vi "Add Items to Graph.vi"(5 "Force Skip? (F)":bool, 7 "Depth Limit (12)":i32=12, 9 "Parent Index (None)":i32=-1, 10 "Items":variant[](array[variant]), 11 "Graph In":T1[](array[typedef])) -> (3 "Graph":T1[](array[typedef]))   [LabVIEW 2016, in "Better Search.lvlib"]
uses:
  Better Search.lvlib
  Data Types/Type Reflection Item.ctl
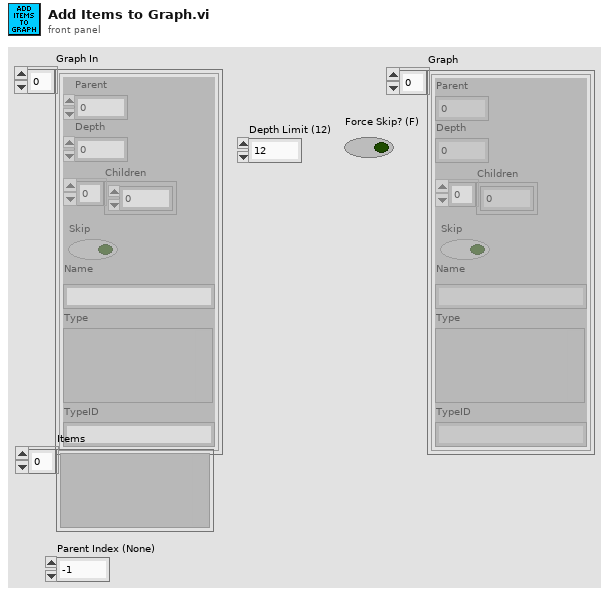
[diagram p1: front panel]
types:
  T1 = typedef "Better Search.lvlib/Type Reflection Item.ctl" = cluster{"Parent":i32, "Depth":i32, "Children":i32[], "Skip":bool, "Name":string, "Type":variant, "TypeID":string}
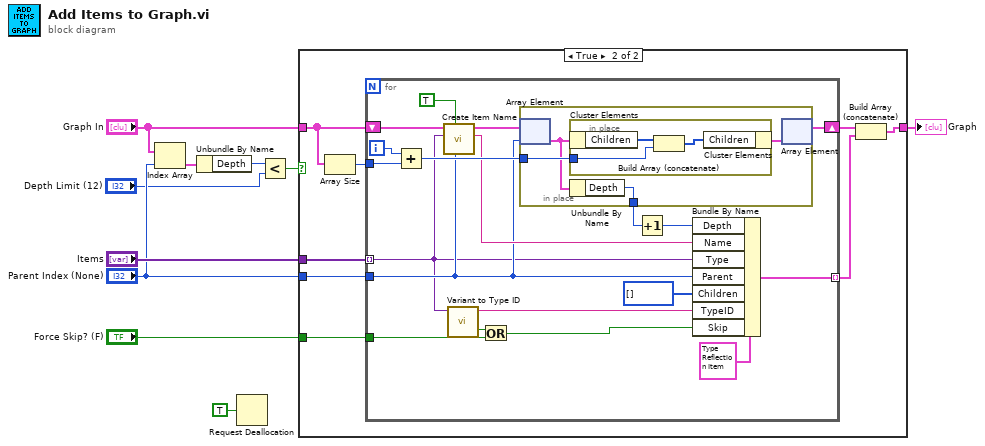
[diagram p0: block diagram]
diagram:
  n1 = Index Array(array="Graph In", index="Parent Index (None)") -> (element=w6:T1)
  n2 = Unbundle By Name(w6) -> ("Depth"=w5:i32)
  n3 = Request Deallocation(TRUE ("flag")) -> ()
  n4 = Less?(x=w5, y="Depth Limit (12)") -> (x < y?=w3:bool)
  n5 = case shown="True" w3 {
    tunnel: [w11 w18] -> w10
    tunnel: "Items" -> [_ w17]
    tunnel: "Graph In" -> [w11 w14]
    tunnel: "Parent Index (None)" -> [_ w13]
    tunnel: "Force Skip? (F)" -> [_ w12]
    frame False {
      # "Already at max depth, don't add more items."
    }
    frame True {
      n6 = Array Size(array=w14) -> (size(s)=w15:i32)
      n7 = for {
        tunnel: w13 -> [w26]
        tunnel: [w37] -> w19 mode=indexing
        tunnel: w17 -> [w23] mode=indexing
        shift-right: [w31] -> w16
        shift-left: w14 -> [w29]
        tunnel: w15 -> [w36]
        tunnel: w12 -> [w20]
        i -> [w35]
        n8 = Add(x=w35, y=w36) -> (x+y=w34:i32)
        n9 = call "Create Item Name.vi"("Parent"=w26, "Hide Full Name? (F)"=TRUE, "Type"=w23, "Item Graph In"=w29) -> ("Name"=w27:string, "Item Graph"=w28:T1[])  [unwired: 6 in]
        n10 = call "Variant to Type ID.vi"("Variant"=w23) -> ("Type ID"=w24:string, "Skip?"=w22:bool)  [unwired: 9 in]
        n11 = Or(x=w22, y=w20) -> (x .or. y?=w21:bool)
        n12 = in-place {
          in-place-border: w34 -> [w42]
          in-place-border: [w39] -> w33
          n13 = in-place-array #1(w28, w26) -> (w40:T1)
          n14 = in-place {
            in-place-border: w42 -> [w44]
            n15 = in-place-cluster #2(w40) -> ("Children"=w45:i32[])
            n16 = Build Array (concatenate)(w45, w44) -> (w43:i32[])
            n17 = in-place-cluster #2("Children"=w43) -> (w41:T1)
          }
          n18 = Unbundle By Name(w40) -> ("Depth"=w39:i32)
          n19 = in-place-array #1(w41) -> (w31:T1[])  [unwired: 1 out]
        }
        n20 = Increment(x=w33) -> (x+1=w30:i32)
        n21 = Bundle By Name(cluster=T1 {"Parent"=-1, "Depth"=0, "Children"=[], "Skip"=FALSE, "Name"="", "Type"=variant, "TypeID"=""} ("Type Reflection Item"), "Depth"=w30, "Name"=w27, "Type"=w23, "Parent"=w26, "Children"=i32[] [], "TypeID"=w24, "Skip"=w21) -> (w37:T1)
      }
      n22 = Build Array (concatenate)(w16, w19) -> (w18:T1[])
    }
  }
  "Graph" <- w10
